vi "Counter - Read Pulse Width and Frequency (On Demand).vi"() -> ()   [LabVIEW 2017]
doc: "本范例演示测量周期、频率、脉冲宽度，本范例演示测量周期、频率、脉冲宽度，或两或两边沿间隔的方法。\n\n本范例不采用缓冲。 由于测量通过软件启动，可能无法采集输入信号信号的每一个周期。 如需确保采集输入的每个周期，可使用“隐式定时”（参考其他计数器输入范例）。\n\n关于将信号连接至DAQ设备的方法，可参考设备文档。"
uses:
  <vilib>/Utility/error.llb/DialogType.ctl
  <vilib>/DAQmx/read.llb/DAQmx Read (Counter DBL 1Chan 1Samp).vi
  <vilib>/DAQmx/create/channels.llb/DAQmx Create Channel (CI-Period).vi
  <vilib>/DAQmx/create/channels.llb/DAQmx Create Channel (CI-Frequency).vi
  <vilib>/DAQmx/create/channels.llb/DAQmx Create Channel (CI-Pulse Width).vi
  <vilib>/DAQmx/create/channels.llb/DAQmx Create Channel (CI-Two Edge Separation).vi
  <vilib>/DAQmx/miscellaneous.llb/DAQmx Fill In Error Info.vi
  <resource>/objmgr/daqmx.rc
panel:
  in  "停止":bool
  out "数据":dbl
  in  "计数器输入类型":T1(tab)
  in  "周期输入接线端":tag="/Dev1/PFI9"
  in  "最大周期":dbl=0.1 format="%0.6f"
  in  "最小周期":dbl=1e-06 format="%0.6f"
  in  "最小频率":dbl=2.0 format="%0.6f"
  in  "最大频率":dbl=100.0 format="%0.6f"
  in  "频率输入接线端":tag="/Dev1/PFI9"
  in  "脉冲宽度输入接线端":tag="/Dev1/PFI9"
  in  "最小脉冲宽度":dbl=1e-06 format="%0.6f"
  in  "最大脉冲宽度":dbl=0.1 format="%0.6f"
  in  "第二个输入信号":tag="/Dev1/PFI9"
  in  "第一个输入接线端":tag="/Dev1/PFI10"
  in  "最小间隔时间":dbl=1e-06 format="%0.6f"
  in  "最大间隔时间":dbl=0.1 format="%0.6f"
  in  "计数器":tag="Dev1/ctr0"
  # "通道设置"
  # "采集数据"
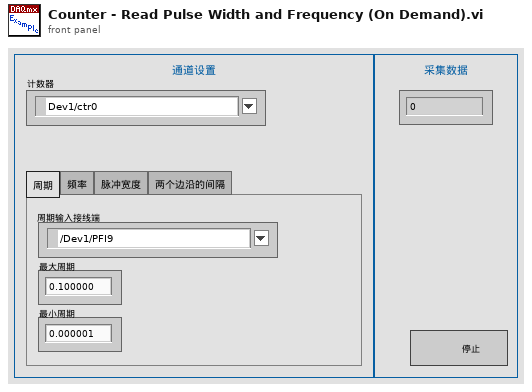
[diagram p1: front panel]
types:
  T1 = enum32{"Period", "Frequency", "Pulse Width", "2 Edge Separation"}
  T2 = typedef "DialogType.ctl" = u16
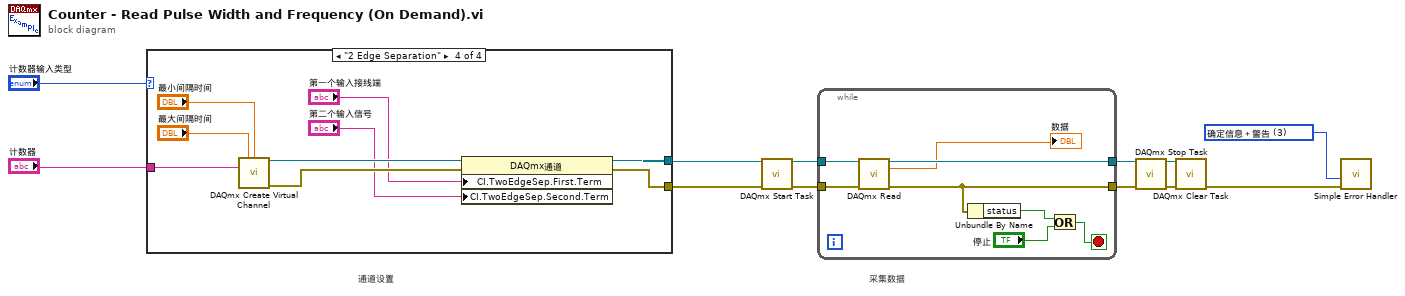
[diagram p0: block diagram]
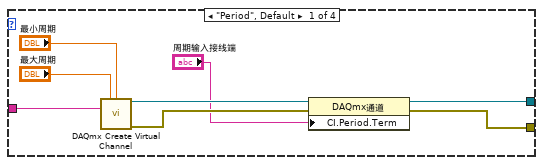
[diagram p2: hidden frame]
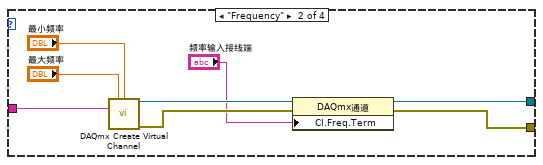
[diagram p3: hidden frame]
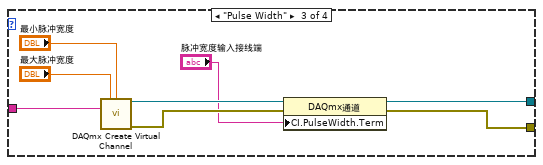
[diagram p4: hidden frame]
diagram:
  w1 = T2 3 items=["无对话框", "确定信息", "继续或停止信息", "确定信息＋警告", "继续/停止＋警告"] ("对话框类型（确定信息：1）")
  # "采集数据"
  # "通道设置"
  n1 = case shown="\"2 Edge Separation\"" "计数器输入类型" {
    tunnel: [w18 w26 w34 w43] -> w7
    tunnel: [w19 w27 w35 w44] -> w6
    tunnel: "计数器" -> [w20 w28 w36 w45]
    frame "Period", Default {
      n2 = call-poly <vilib>:"DAQmx Create Virtual Channel.vi"("maximum value"="最大周期", "minimum value"="最小周期", "counter"=w20) -> ("task out"=w17:refnum<k21>, "error out"=w16:errorcluster)  [unwired: 11 in]
      n3 = property class="DAQmx通道"(reference=w17, error in=w16, "CI.Period.Term"="周期输入接线端") -> (reference out=w19:refnum<k21>, error out=w18:errorcluster)
    }
    frame "Frequency" {
      n4 = call-poly <vilib>:"DAQmx Create Virtual Channel.vi"("maximum value"="最大频率", "minimum value"="最小频率", "counter"=w28) -> ("task out"=w25:refnum<k21>, "error out"=w24:errorcluster)  [unwired: 11 in]
      n5 = property class="DAQmx通道"(reference=w25, error in=w24, "CI.Freq.Term"="频率输入接线端") -> (reference out=w27:refnum<k21>, error out=w26:errorcluster)
    }
    frame "Pulse Width" {
      n6 = call-poly <vilib>:"DAQmx Create Virtual Channel.vi"("maximum value"="最大脉冲宽度", "minimum value"="最小脉冲宽度", "counter"=w36) -> ("task out"=w33:refnum<k21>, "error out"=w32:errorcluster)  [unwired: 11 in]
      n7 = property class="DAQmx通道"(reference=w33, error in=w32, "CI.PulseWidth.Term"="脉冲宽度输入接线端") -> (reference out=w35:refnum<k21>, error out=w34:errorcluster)
    }
    frame "2 Edge Separation" {
      n8 = call-poly <vilib>:"DAQmx Create Virtual Channel.vi"("maximum value"="最大间隔时间", "minimum value"="最小间隔时间", "counter"=w45) -> ("task out"=w42:refnum<k21>, "error out"=w41:errorcluster)  [unwired: 11 in]
      n9 = property class="DAQmx通道"(reference=w42, error in=w41, "CI.TwoEdgeSep.First.Term"="第一个输入接线端", "CI.TwoEdgeSep.Second.Term"="第二个输入信号") -> (reference out=w44:refnum<k21>, error out=w43:errorcluster)
    }
  }
  n10 = call <vilib>:"DAQmx Start Task.vi"("task/channels in"=w6, "error in"=w7) -> ("task out"=w12:refnum<k21>, "error out"=w11:errorcluster)  [unwired: 12 in]
  n11 = while {
    tunnel: w12 -> [w53]
    tunnel: w11 -> [w52]
    tunnel: [w51] -> w2
    tunnel: [w49] -> w3
    stop <- w46 stop-if-true
    n12 = call-poly <vilib>:"DAQmx Read.vi"("task/channels in"=w53, "error in"=w52) -> ("task out"=w51:refnum<k21>, "data"=→"数据":dbl, "error out"=w49:errorcluster)  [unwired: 11 in]
    n13 = Unbundle By Name(w49) -> ("status"=w48:bool)
    n14 = Or(x=w48, y="停止") -> (x .or. y?=w46:bool)
  }
  n15 = call <vilib>:"DAQmx Stop Task.vi"("task/channels in"=w2, "error in"=w3) -> ("task out"=w5:refnum<k21>, "error out"=w4:errorcluster)  [unwired: 12 in]
  n16 = call <vilib>:"DAQmx Clear Task.vi"("task in"=w5, "error in"=w4) -> ("error out"=w10:errorcluster)  [unwired: 13 in]
  n17 = call <vilib>:"Simple Error Handler.vi"("type of dialog (OK msg:1)"=w1, "error in (no error)"=w10) -> ()  [unwired: 3 in, 5 out]
